vi "Read Boolean.vi"(7 "section":string, 8 "error in":errorcluster, 9 "default value":bool, 10 "key":string, 11 "config file in":refnum<data-value>) -> (0 "error out":errorcluster, 1 "value":bool, 2 "found?":bool, 3 "config file out":refnum<data-value>)   [LabVIEW 2012, in "configlib.lvlib"]
uses:
  configlib.lvlib
  Configuration File Definition.ctl
  File Options.ctl
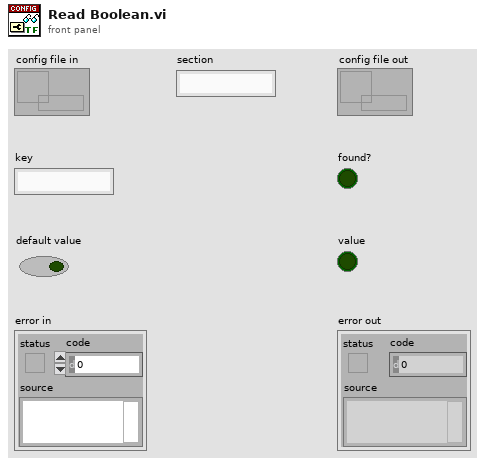
[diagram p1: front panel]
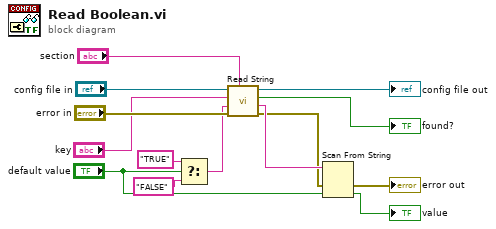
[diagram p0: block diagram]
diagram:
  n1 = Select(t="TRUE" ("resulting string 2"), s="default value", f="FALSE" ("resulting string 2")) -> (s? t:f=w9:string)
  n2 = call "Read String.vi"("section"="section", "error in"="error in", "default"=w9, "key"="key", "config file in"="config file in") -> ("error out"=w3:errorcluster, "value"=w5:string, "found?"=→"found?":bool, "config file out"=→"config file out":refnum<data-value>)  [unwired: 3 in]
  n3 = Scan From String(input string=w5, error in=w3, default 1="default value") -> (error out=→"error out":errorcluster, output 1=→"value":bool)  [unwired: 2 in, 2 out]
